vi "Select Menu Dialog box.vi"(9 "Starting index":i32, 10 "Message in":string, 11 "Options in":string[](array[string])) -> (2 "Selected option number":i32)   [LabVIEW 2025, in "MyLockIn.lvlib"]
uses:
  MyLockIn.lvlib
panel:
  in  "WC instrument menu":string(combo) caption="Select option"
  in  "stop":bool
  out "Show message":string
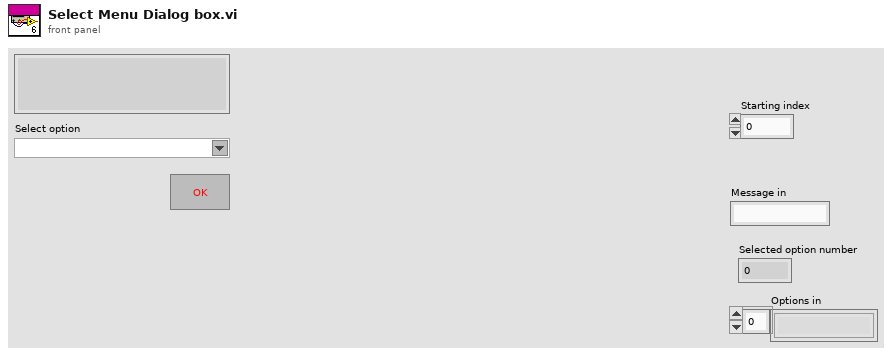
[diagram p1: front panel]
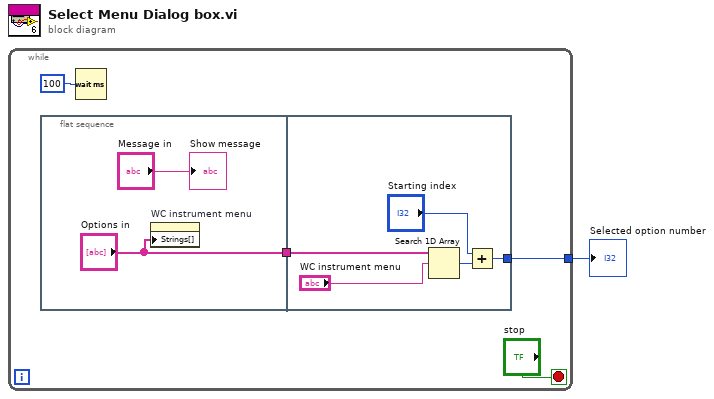
[diagram p0: block diagram]
diagram:
  n1 = while {
    tunnel: [w4] -> w1
    stop <- "stop" stop-if-true
    n2 = flat-sequence {
      tunnel: ["Options in"] -> w2
      tunnel: [w9] -> w4
      tunnel: w2 -> [w11]
      frame #0 {
        n3 = property on="WC instrument menu" class="CmbBox"("Strings[]"="Options in") -> ()  [unwired: 2 in, 2 out]
        "Show message" <- "Message in"
      }
      frame #1 {
        n4 = Search 1D Array(1D array=w11, element="WC instrument menu") -> (index of element=w10:i32)  [unwired: 1 in]
        n5 = Add(x="Starting index", y=w10) -> (x+y=w9:i32)
      }
    }
    n6 = Wait (ms)(milliseconds to wait=u32 100) -> ()  [unwired: 1 out]
  }
  "Selected option number" <- w1
